vi "GetLeCroy_PassData.vi"(1 "lines per plane":i32, 5 "File Array":string[](array[string]), 7 "Digitizer Settings":T1={"Digitizer delay (us) "=0.0, "rf points per line"=2048, "lines per plane"=128, "Samp Rate (Hz)"=100000000.0, "Additional dig delay (us)"=0.0, "Voltage Scale"=0.4, "Pre-Looks"=0, "Offset delay (us)"=0.0, "bits A/D"=8, "Avg Num"=1, "DigTimeOut"=5.0, "Rel Dig Delay"=0.0, "Dig Ch"=0, "LeCroyCluster"={"LeCroy Channels"=[TRUE, FALSE, FALSE, FALSE], "LC read pt offset"=0.0, "Sweep Avg"=FALSE}, "Main Digitizer"=enum."NI Digitizer", "Dig Config"=enum."Single channel", "Digitizer ID Cluster"={"Acqiris/Alazar/SP ID"=[], "NI Instr Handles"=[], "LeCroy VISA"="", "GaGe Handle"={"Handle"=0, "Sample size"=0, "Resolution"=0, "Offset"=0, "Channels"=0, "Boards"=0}, "ATS Ref"="ATS9350", "Acqiris Address"=["PCI::INSTR0"], "ADQRef"=refnum, "adq_cu_ptr"=refnum}, "Trigger Settings"={"Trig Source"=1, "Trig Coupling"=0, "Trig Slope"=0, "Level (mV)"=1500.0}, "Bulk Acq"=FALSE, "Bulk Start Indexes"=[], "Data Ref RF"=refnum, "NI ID/Channel"=[], "Total Dig CH"=1, "Xtra Ann Trig delay (us)"=10.0, "Fix Z Delay?"=FALSE, "One Way Transmission?"=FALSE, "Data Ref Log"=refnum} {"Trigger Settings"."Trig Slope" items=["Positive", "Negative"]; "Trigger Settings"."Level (mV)" format="%.2f"; "Trigger Settings"."Trig Coupling" items=["DC 1 MOhm", "AC 1 MOhm", "DC 50 Ohm", "AC 50 Ohm"]; "Trigger Settings"."Trig Source" items=["Chan 1", "External"]; "Rel Dig Delay" format="%.2f"; "DigTimeOut" format="%.2f"; "Avg Num" min=1; "Offset delay (us)" format="%.2f"; "Additional dig delay (us)" format="%.2f"; "Digitizer delay (us)" format="%.2f"}, 11 "error in":errorcluster, 13 "Reverse?":bool) -> (3 "VGain (dB)":dbl, 6 "Gain Array":T6(array[cluster]), 8 "Array out":i16[][][](array[numeric]), 14 "Raw VGain (scale)":dbl, 15 "error out":errorcluster)   [LabVIEW 2022 SP3]
uses:
  -DigitizerRoutines/DigitizerSettings.ctl
  -DigitizerRoutines/Digitizer.ctl
  -DigitizerRoutines/DigConfig.ctl
  -DigitizerRoutines/DigitizerID.ctl
  C:/Windows/System32/ADQAPI_dotNet_helper.dll
  -ScanSystem/DataHandling/ReverseData.vi
panel:
  out "Voltage Scale":T5
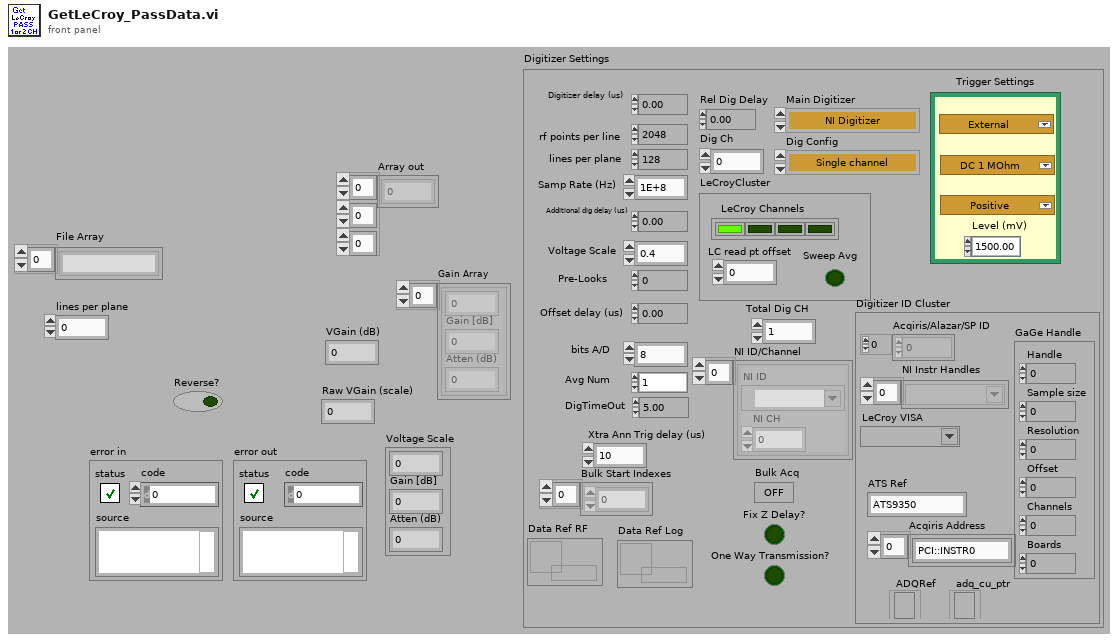
[diagram p1: front panel]
types:
  T1 = typedef "DigitizerSettings.ctl" = cluster{"Digitizer delay (us) ":dbl, "rf points per line":i32, "lines per plane":i32, "Samp Rate (Hz)":dbl, "Additional dig delay (us)":dbl, "Voltage Scale":dbl, "Pre-Looks":i32, "Offset delay (us)":dbl, "bits A/D":i8, "Avg Num":i32, "DigTimeOut":sgl, "Rel Dig Delay":sgl, "Dig Ch":i32, "LeCroyCluster":cluster{"LeCroy Channels":bool[], "LC read pt offset":dbl, "Sweep Avg":bool}, "Main Digitizer":T2, "Dig Config":T3, "Digitizer ID Cluster":T4, "Trigger Settings":cluster{"Trig Source":u16, "Trig Coupling":u16, "Trig Slope":u16, "Level (mV)":dbl}, "Bulk Acq":bool, "Bulk Start Indexes":i32[], "Data Ref RF":refnum<data-value>, "NI ID/Channel":cluster{"NI ID":refnum<k15>, "NI CH":i32}[], "Total Dig CH":i32, "Xtra Ann Trig delay (us)":dbl, "Fix Z Delay?":bool, "One Way Transmission?":bool, "Data Ref Log":refnum<data-value>}
  T2 = typedef "Digitizer.ctl" = enum16{"Acqiris Digitizer", "NI Digitizer", "LeCroy", "GaGe", "AlazarTech", "No Digitizer", "Teledyne"}
  T3 = typedef "DigConfig.ctl" = enum16{"Single channel", "2 Chans w/ 2 Acqiris", "2 Chans w/ 1 Acqiris", "5-CH Pulser New", "5-CH pulser w/ ann array", "5-pass style ann array", "Empty"}
  T4 = typedef "DigitizerID.ctl" = cluster{"Acqiris/Alazar/SP ID":u32[], "NI Instr Handles":refnum<k15>[], "LeCroy VISA":refnum<visa-resource-name>, "GaGe Handle":cluster{"Handle":u32, "Sample size":u32, "Resolution":i32, "Offset":i32, "Channels":u32, "Boards":u32}, "ATS Ref":string, "Acqiris Address":string[], "ADQRef":refnum<k24>, "adq_cu_ptr":refnum<k24>}
  T5 = cluster{sgl, "Gain [dB]  ":sgl, "Atten (dB)":sgl}
  T6 = cluster{sgl, "Gain [dB]  ":sgl, "Atten (dB)":sgl}[]
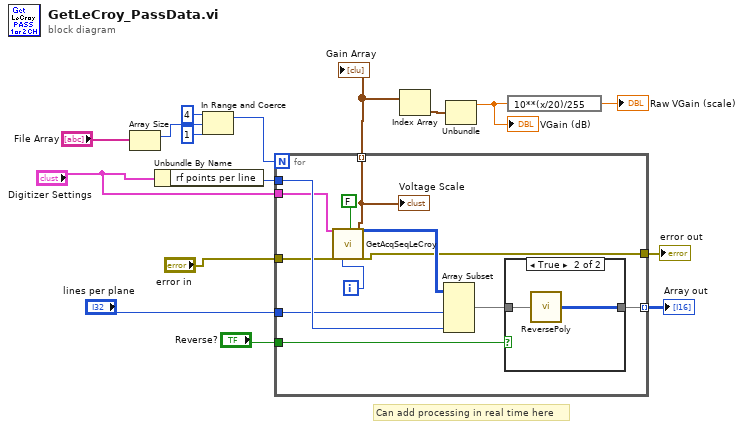
[diagram p0: block diagram]
diagram:
  # "Can add processing in real time here"
  n1 = Array Size(array="File Array") -> (size(s)=w4:i32)
  n2 = Unbundle By Name("Digitizer Settings") -> ("rf points per line"=w7:i32)
  n3 = In Range and Coerce(upper limit=4, x=w4, lower limit=1) -> (coerced(x)=w2:i32)  [unwired: 1 out]
  n4 = for {
    N: w2 -> [_]
    tunnel: w7 -> [w28]
    tunnel: "lines per plane" -> [w27]
    tunnel: "Reverse?" -> [w26]
    tunnel: [w24] -> w8 mode=indexing
    tunnel: [w20] -> w6
    tunnel: "error in" -> [w19]
    tunnel: "Digitizer Settings" -> [w18]
    tunnel: [w17] -> w9 mode=indexing
    i -> [w22]
    n5 = call "GetAcqSeqLeCroy.vi"("Digitizer Settings"=w18, "errorin"=w19, "Source (0: Channel 1)"=w22, "save?"=FALSE) -> ("Voltage Scale"=w17:T5, "Data Array"=w23:i16[][], "error out"=w20:errorcluster)  [unwired: 17 in, 4 out]
    "Voltage Scale" <- w17
    n6 = Array Subset(array=w23, length (row)=w27, length (col)=w28) -> (w25:i16[][])  [unwired: 2 in]
    n7 = case shown="True" w26 {
      tunnel: [w29 w31] -> w24
      tunnel: w25 -> [w29 w30]
      frame False {
      }
      frame True {
        n8 = call-poly "ReversePoly.vi"("Array in"=w30) -> ("Array out"=w31:i16[][])
      }
    }
  }
  "Gain Array" <- w9
  "Array out" <- w8
  "error out" <- w6
  n9 = Index Array(array=w9) -> (element=w10:T5)  [unwired: 1 in]
  n10 = Unbundle(w10) -> (w11:sgl)  [unwired: 2 out]
  "VGain (dB)" <- w11
  n11 = expression code="10**(x/20)/255"(w11) -> (→"Raw VGain (scale)":sgl)
